vi "BeeHarmonicRadar.vi"(4 "Negates for Encoders":cluster{"Right Negate":bool, "Left Negate":bool}, 6 "Sampling Period":u32=10, 7 "Encoder Velocity Configuration":T1={"Right Encoder Rate to Velocity"=1.0, "Left Encoder Rate to Velocity"=1.0}, 8 "Reckoned Position FIFO Name":string="Position", 9 "Yaw RT FIFO":string="Yaw", 10 "Initial Values":T7, 11 "Encoder Dev Refs":T6={"RightEncoderDevRef"={"DevStatus"={"status"=FALSE, "code"=0, "source"=""}, "EncoderIndex"=enum."Invalid", "CounterIndex"=enum."Invalid", "DistancePerCount"=1.0, "Decoding Type"=enum."4x"}, "LeftEncoderDevRef"={"DevStatus"={"status"=FALSE, "code"=0, "source"=""}, "EncoderIndex"=enum."Invalid", "CounterIndex"=enum."Invalid", "DistancePerCount"=1.0, "Decoding Type"=enum."4x"}}) -> ()   [LabVIEW 2016]
uses:
  <vilib>/Rock Robotics/WPI/Encoder/WPI_EncoderDevRef.ctl
  <vilib>/Rock Robotics/SystemInterfaces/Encoder/FPGA_EncoderIdx.ctl
  <vilib>/Rock Robotics/SystemInterfaces/Counter/FPGA_CounterCtrSystemIndex.ctl
  <vilib>/Rock Robotics/WPI/Encoder/WPI_EncoderType.ctl
  <vilib>/Platform/TimedLoop/XDataNode/timing_clust.ctl
  <vilib>/Platform/TimedLoop/XDataNode/nitl_modes.ctl
  <vilib>/Platform/TimedLoop/XDataNode/wakeup.ctl
  <vilib>/platform/TimedLoop/XDataNode/XDataNode.xnode
  <vilib>/Platform/TimedLoop/XDataNode/XDNodeRunTimeDep.lvlib
panel:
  out "Y Trap + Gyro":dbl
  out "X Trap + Gyro":dbl
  in  "Reset":bool
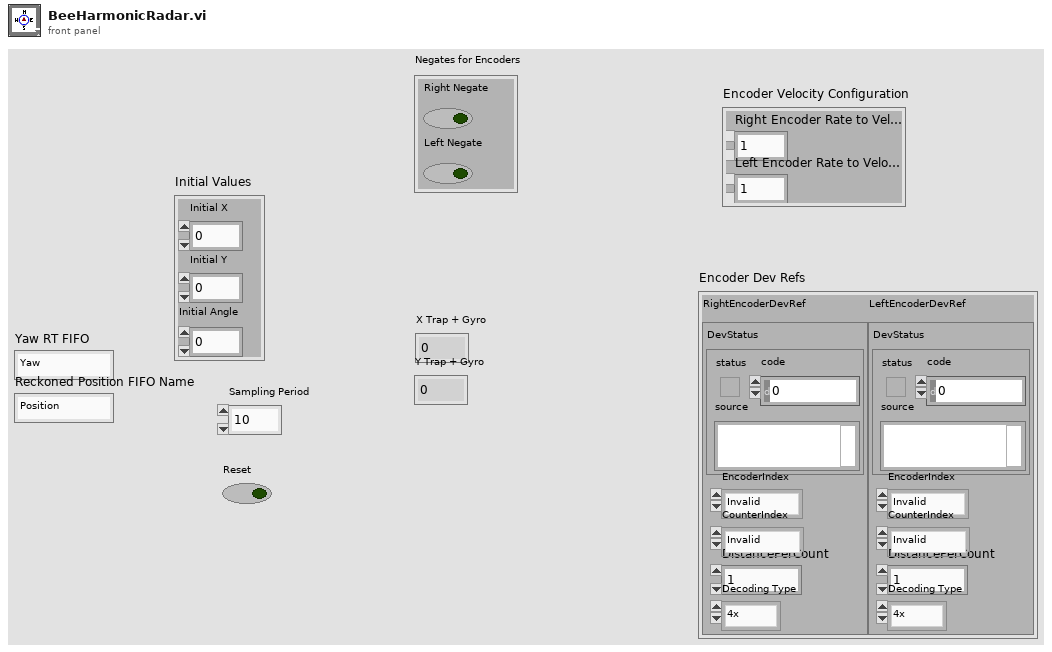
[diagram p1: front panel]
types:
  T1 = cluster{"Right Encoder Rate to Velocity":dbl, "Left Encoder Rate to Velocity":dbl}
  T2 = typedef "WPI_EncoderDevRef.ctl" = cluster{"DevStatus":errorcluster, "EncoderIndex":T3, "CounterIndex":T4, "DistancePerCount":dbl, "Decoding Type":T5}
  T3 = typedef "FPGA_EncoderIdx.ctl" = enum8{"Enc 0", "Enc 1", "Enc 2", "Enc 3", "Enc 4", "Enc 5", "Enc 6", "Enc 7", "Invalid"}
  T4 = typedef "FPGA_CounterCtrSystemIndex.ctl" = enum8{"Ctr 0", "Ctr 1", "Ctr 2", "Ctr 3", "Ctr 4", "Ctr 5", "Ctr 6", "Ctr 7", "Invalid"}
  T5 = typedef "WPI_EncoderType.ctl" = enum16{"1x", "2x", "4x"}
  T6 = cluster{"RightEncoderDevRef":T2, "LeftEncoderDevRef":T2}
  T7 = cluster{"Initial X":dbl, "Initial Y":dbl, "Initial Angle":dbl}
  T8 = typedef "XDNodeRunTimeDep.lvlib/timing_clust.ctl" = cluster{"Expected End [f-1]":u64, "Actual End [f-1]":u64, "Finished Late? [f-1]":bool, "Expected End [i-1]":u64, "Actual End [i-1]":u64, "Finished Late? [i-1]":bool, "Expected Start [i]":u64, "Actual Start [i]":u64, "Expected Start [f]":u64, "Actual Start [f]":u64, "Source Name":string, "Structure Name":string, "Period":i64, "Deadline":i64, "Offset":i64, "Start":i64, "Priority":i32, "Timeout":i32, "Mode":T9, "Wakeup Reason":T10, "Error":errorcluster, "Source Type":string, "Secondary Source Type":string, "Global End Time":u64, "Global Start Time":u64, "Frame Duration":u64, "Iteration Duration":u64, "Assigned CPU":i32, "I/O Scan Engine Mode":u32}
  T9 = typedef "XDNodeRunTimeDep.lvlib/nitl_modes.ctl" = enum32{"No Change", "Process missed periods, maintain original phase", "Discard missed periods, maintain original phase", "Process missed periods, ignore original phase", "Discard missed periods, ignore original phase"}
  T10 = typedef "XDNodeRunTimeDep.lvlib/wakeup.ctl" = enum32{"Normal", "Aborted", "Asynchronous wakeup", "Timing source error", "Timed loop error", "Timeout"}
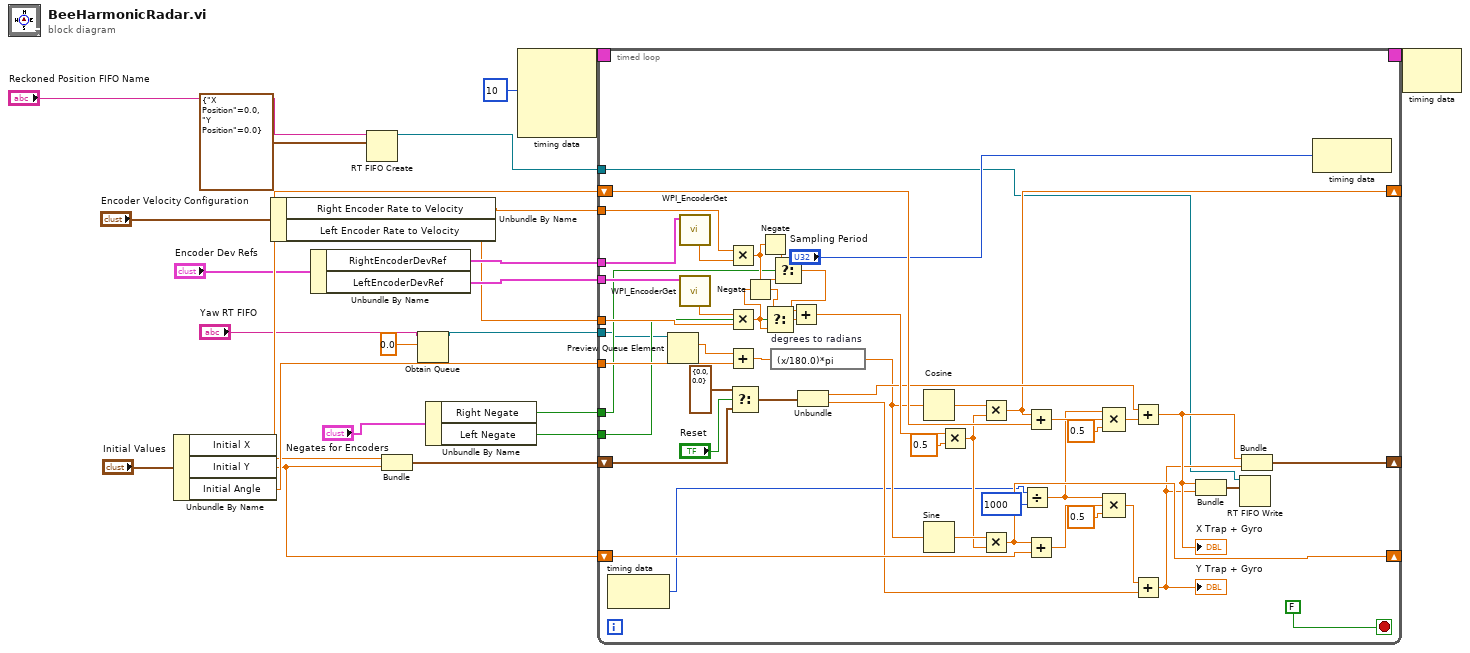
[diagram p0: block diagram]
diagram:
  n1 = Unbundle By Name("Initial Values") -> ("Initial X"=w13:dbl, "Initial Y"=w14:dbl, "Initial Angle"=w15:dbl)
  n2 = Unbundle By Name("Encoder Velocity Configuration") -> ("Right Encoder Rate to Velocity"=w8:dbl, "Left Encoder Rate to Velocity"=w7:dbl)
  n3 = Unbundle By Name("Encoder Dev Refs") -> ("RightEncoderDevRef"=w11:T2, "LeftEncoderDevRef"=w10:T2)
  n4 = RT FIFO Create(0:"Reckoned Position FIFO Name", 1:cluster{"X Position":dbl, "Y Position":dbl} {"X Position"=0.0, "Y Position"=0.0}) -> (8:w17:refnum<k33>)  [unwired: 6 in, 2 out]
  n5 = Bundle("Initial X"=w13, "Initial Y"=w14) -> (w23:cluster{"Initial X":dbl, "Initial Y":dbl})  [unwired: 1 in]
  n6 = Obtain Queue(name (unnamed)="Yaw RT FIFO", element data type=0.0) -> (queue out=w2:refnum<queue>)  [unwired: 3 in, 2 out]
  n7 = Unbundle By Name("Negates for Encoders") -> ("Right Negate"=w5:bool, "Left Negate"=w4:bool)
  n8 = node-c288(i64 10 ("Period")) -> (w22:T8)  [unwired: 3 in]
  n9 = timed-loop {
    tunnel: w15 -> [w72]
    shift-right: [w56] -> _
    shift-left: w14 -> [w70]
    shift-right: [w53] -> _
    shift-left: w13 -> [w69]
    shift-right: [w60] -> _
    shift-left: w23 -> [w45]
    timing: w22 -> [_]
    timing-out: [_] -> w21
    tunnel: w10 -> [w52]
    tunnel: w11 -> [w51]
    tunnel: w2 -> [w25]
    tunnel: w17 -> [w38]
    tunnel: w8 -> [w37]
    tunnel: w7 -> [w36]
    tunnel: w5 -> [w33]
    tunnel: w4 -> [w28]
    stop <- FALSE stop-if-true
    n10 = node-c288() -> (w27:i64)  [unwired: 1 in]
    n11 = Preview Queue Element(queue=w25) -> (element=w24:dbl)  [unwired: 2 in, 3 out]
    n12 = call <vilib>:"WPI_EncoderGet.vi"("EncoderDevRef"=w51) -> ("Rate"=w43:dbl)  [unwired: 5 in, 5 out]
    n13 = call <vilib>:"WPI_EncoderGet.vi"("EncoderDevRef"=w52) -> ("Rate"=w42:dbl)  [unwired: 5 in, 5 out]
    n14 = Multiply(x=w37, y=w43) -> (x*y=w35:dbl)
    n15 = Multiply(x=w42, y=w36) -> (x*y=w30:dbl)
    n16 = Add(x=w24, y=w72) -> (x+y=w71:dbl)
    n17 = Select(t=cluster{"Initial X":dbl, "Initial Y":dbl} {"Initial X"=0.0, "Initial Y"=0.0}, s="Reset", f=w45) -> (s? t:f=w44:cluster{"Initial X":dbl, "Initial Y":dbl})
    n18 = Negate(x=w30) -> (-x=w29:dbl)
    n19 = Negate(x=w35) -> (-x=w34:dbl)
    n20 = Select(t=w29, s=w28, f=w30) -> (s? t:f=w31:dbl)
    n21 = expression code="(x/180.0)*pi" "degrees to radians"(w71) -> (w48:dbl)
    n22 = Select(t=w34, s=w33, f=w35) -> (s? t:f=w32:dbl)
    n23 = Add(x=w32, y=w31) -> (x+y=w68:dbl)
    n24 = Unbundle(w44) -> ("Initial X"=w59:dbl, "Initial Y"=w58:dbl)
    n25 = Cosine(x=w48) -> (cos(x)=w54:dbl)
    n26 = Sine(x=w48) -> (sin(x)=w57:dbl)
    n27 = Multiply(x=w68, y=0.5) -> (x*y=w55:dbl)
    n28 = Multiply(x=w54, y=w55) -> (x*y=w53:dbl)
    n29 = Multiply(x=w57, y=w55) -> (x*y=w56:dbl)
    n30 = Divide(x=w27, y=u32 1000) -> (x/y=w50:dbl)
    n31 = Add(x=w53, y=w69) -> (x+y=w65:dbl)
    n32 = Add(x=w56, y=w70) -> (x+y=w63:dbl)
    n33 = Compound Arithmetic op=MULTIPLY(w50, w65, 0.5 ("y")) -> (w62:dbl)
    n34 = Compound Arithmetic op=MULTIPLY(w50, w63, 0.5 ("y")) -> (w61:dbl)
    n35 = Add(x=w59, y=w62) -> (x+y=w41:dbl)
    "X Trap + Gyro" <- w41
    n36 = Add(x=w61, y=w58) -> (x+y=w40:dbl)
    "Y Trap + Gyro" <- w40
    n37 = Bundle(w41, w40) -> (w39:cluster{dbl, dbl})  [unwired: 1 in]
    n38 = RT FIFO Write(0:w38, 1:w39) -> ()  [unwired: 3 in, 4 out]
    n39 = Bundle(w41, w40) -> (w60:cluster{dbl, dbl})  [unwired: 1 in]
    n40 = node-c288("Sampling Period") -> ()  [unwired: 1 out]
  }
  n41 = node-c288(w21) -> ()  [unwired: 1 out]
